vi "niRFUtil WFM Interpolate Waveform (complex wfm).vi"(0 "Waveform In":T1 {"y" format="%.2f"; "dx" format="%^.2e"; "x0" format="%^.2e"}, 5 "Rate (1)":i32=1, 7 "Offset (0)":i32) -> (4 "Waveform Out":T1 {"y" format="%.2f"; "dx" format="%^.2e"; "x0" format="%^.2e"})   [LabVIEW 2015, in "niRFUtil.lvlib"]
doc: "(c) Copyright 2006, National Instruments, Inc. This VI may not be duplicated, sold, or distributed without written consent from National Instruments."
uses:
  niRFUtil.lvlib
  Includes/niRFUtil INC Complex Waveform.ctl
  Includes/niRFUtil INC Complex Array.ctl
  <vilib>/Analysis/2dsp.llb/Upsample (CDB).vi
  <vilib>/Analysis/NI_AALPro.lvlib
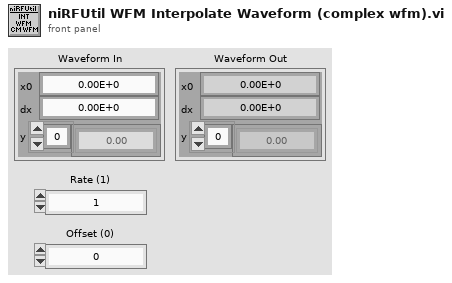
[diagram p1: front panel]
types:
  T1 = typedef "niRFUtil.lvlib/niRFUtil INC Complex Waveform.ctl" = cluster{"x0":dbl, "dx":dbl, "y":T2}
  T2 = typedef "niRFUtil.lvlib/niRFUtil INC Complex Array.ctl" = csg[]
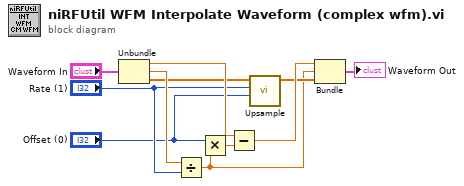
[diagram p0: block diagram]
diagram:
  n1 = Unbundle("Waveform In") -> ("x0"=w9:dbl, "dx"=w11:dbl, "y"=w7:T2)
  n2 = Divide(x=w11, y="Rate (1)") -> (x/y=w5:dbl)
  n3 = Multiply(x="Offset (0)", y=w5) -> (x*y=w10:dbl)
  n4 = Subtract(x=w9, y=w10) -> (x-y=w8:dbl)
  n5 = call-poly <vilib>:"Upsample.vi"("leading zeros"="Offset (0)", "upsampling factor"="Rate (1)", "X"=w7) -> ("Upsampled Array"=w6:cdb[])  [unwired: 8 out]
  n6 = Bundle(w8, w5, "Upsampled Array"=w6) -> (→"Waveform Out":cluster{dbl, dbl, "Upsampled Array":cdb[]})  [unwired: 1 out]
